vi "PI2_AAN.vi"() -> ()   [LabVIEW 2016]
uses:
  <vilib>/Platform/TimedLoop/XDataNode/nitl_modes.ctl
  <vilib>/Platform/TimedLoop/XDataNode/XDNodeRunTimeDep.lvlib
  <vilib>/Platform/TimedLoop/XDataNode/XDataNode.xnode
  <vilib>/Platform/TimedLoop/XDataNode/timing_clust.ctl
  <vilib>/Platform/TimedLoop/XDataNode/wakeup.ctl
  <vilib>/imath/engines/lvmath2/RunTimeEngine/NodeEndStatement/NIMS_NodeEndStatement_Output.vi
  <vilib>/imath/engines/lvmath2/RunTimeEngine/ErrorHandling/NIMS_Finalize Error.vi
  <vilib>/imath/engines/lvmath2/RunTimeEngine/Managers/WorkSpace/UID Generator.vi
  <vilib>/imath/engines/lvmath2/RunTimeEngine/ArithmeticOperatorToken/NIMS_ArithmeticOperator_times.vi
  <vilib>/imath/engines/lvmath2/RunTimeEngine/BuiltInFunctions/sum/NIMS_sum(GV).vi
  <vilib>/imathl/engines/lvmath/Functions/Error Handling/Create Error.vi
  <vilib>/imath/engines/lvmath2/RunTimeEngine/RangeToken/NIMS_Range.vi
  <vilib>/imath/engines/lvmath2/RunTimeEngine/ArithmeticOperatorToken/NIMS_ArithmeticOperator_plus.vi
  <vilib>/imath/engines/lvmath2/RunTimeEngine/ErrorHandling/NIMS_Create Error From Enums.vi
  <vilib>/imath/engines/lvmath2/RunTimeEngine/BuiltInFunctions/mod/NIMS_mod_no_size_check.vi
  <vilib>/imath/engines/lvmath2/RunTimeEngine/IndexRead/NIMS V(S).vi
  <vilib>/imath/engines/lvmath2/RunTimeEngine/LocalVariableDefStatement/MC_LocalVariableDefStatement_Display.vi
  <vilib>/imath/engines/lvmath2/RunTimeEngine/RunTimeType/NIMS_RunTimeType_From StrictType (excl LVString).vi
  <vilib>/imath/engines/lvmath2/RunTimeEngine/BuiltInFunctions/linramp/NIMS_linramp.vi
  <vilib>/imath/engines/lvmath2/RunTimeEngine/BuiltInFunctions/eye/NIMS_M=eye(I32).vi
  <vilib>/imath/engines/lvmath2/RunTimeEngine/ErrorHandling/NIMS_Error From Error Code.vi
  <vilib>/imath/engines/lvmath2/RunTimeEngine/BuiltInFunctions/zeros/NIMS_V=zeros(I32,I32).vi
  <vilib>/imath/engines/lvmath2/RunTimeEngine/BuiltInFunctions/zeros/NIMS_M=zeros(I32,I32).vi
  <vilib>/imath/engines/lvmath2/RunTimeEngine/IndexReplace/NIMS V(S)=S.vi
  <vilib>/imath/engines/lvmath2/RunTimeEngine/IndexRead/NIMS V(R2).vi
  <vilib>/imath/engines/lvmath2/RunTimeEngine/RangeToken/NIMS_Range_R2 - Float.vi
  <vilib>/imath/engines/lvmath2/RunTimeEngine/IndexRead/NIMS V(V).vi
  <vilib>/imath/engines/lvmath2/RunTimeSupport/NIMS_Error if Not Equal.vi
  <vilib>/imath/engines/lvmath2/RunTimeEngine/ArithmeticOperatorToken/NIMS_ArithmeticOperator_minus.vi
  <vilib>/imath/engines/lvmath2/RunTimeEngine/ArithmeticOperatorToken/NIMS_ArithmeticOperator_power(S).vi
  <vilib>/imath/engines/lvmath2/RunTimeEngine/BuiltInFunctions/abs/NIMS_abs(signed).vi
  <vilib>/imath/engines/lvmath2/RunTimeEngine/CommandStatement/MC_CommandStatement_break.vi
  <vilib>/imath/engines/lvmath2/RunTimeEngine/IndexRead/NIMS M($,S).vi
  <vilib>/imath/engines/lvmath2/RunTimeEngine/IndexReplace/NIMS M($,S)=V.vi
  <vilib>/imath/engines/lvmath2/RunTimeEngine/ArithmeticOperatorToken/NIMS_ArithmeticOperator_multmx(M,CV).vi
  <vilib>/imath/engines/lvmath2/RunTimeEngine/ArithmeticOperatorToken/NIMS_ArithmeticOperator_multmx.vi
  <vilib>/imath/engines/lvmath2/RunTimeEngine/BuiltInFunctions/randnormal/NIMS_randnormal().vi
  <vilib>/imath/engines/lvmath2/RunTimeEngine/BuiltInFunctions/rand/NIMS_rand().vi
  <vilib>/imath/engines/lvmath2/RunTimeEngine/IndexRead/NIMS M($,V).vi
  <vilib>/imath/engines/lvmath2/RunTimeEngine/BuiltInFunctions/sum/NIMS_sum(GM,Sca).vi
  <vilib>/imath/engines/lvmath2/RunTimeEngine/IndexRead/NIMS M(S,S).vi
  <vilib>/imath/engines/lvmath2/RunTimeEngine/IndexReplace/NIMS M($,S)=M.vi
  <vilib>/imath/engines/lvmath2/RunTimeEngine/VariableToken/Support/NIMS_Scalar Boolean Index to I32 Index.vi
  <vilib>/imath/engines/lvmath2/RunTimeEngine/BuiltInFunctions/randnormal/NIMS_randnormal(1,I32).vi
  <vilib>/imath/engines/lvmath2/RunTimeEngine/VariableToken/NIMS_VariableToken_CondDefined.vi
  <vilib>/imath/engines/lvmath2/RunTimeEngine/Managers/SymbolTable/Clear UID.vi
  <vilib>/imath/engines/lvmath2/RunTimeEngine/Managers/SymbolTable/NIMS_WorkSpace.lvlib
  <vilib>/imath/engines/lvmath/Functions/Error Handling/MergeErrorsWrapper.vi
  <vilib>/imath/engines/lvmath2/RunTimeEngine/IndexReplace/NIMS V(V)=S.vi
  <vilib>/imath/engines/lvmath2/RunTimeEngine/IndexReplace/NIMS V(S)=V.vi
  <vilib>/imath/engines/lvmath2/RunTimeEngine/ArithmeticOperatorToken/NIMS_ArithmeticOperator_rightdiv(C,C).vi
  <vilib>/imath/engines/lvmath2/RunTimeEngine/BuiltInFunctions/min/1 input/NIMS_min(CV).vi
  <vilib>/imath/engines/lvmath2/RunTimeEngine/BuiltInFunctions/max/1 input/NIMS_max(CM).vi
  <vilib>/imath/engines/lvmath2/RunTimeEngine/BuiltInFunctions/max/1 input/NIMS_max(CV).vi
  <vilib>/imath/engines/lvmath2/RunTimeEngine/BuiltInFunctions/min/1 input/NIMS_min(CM).vi
  <vilib>/imath/engines/lvmath2/RunTimeEngine/IndexReplace/NIMS M($,S)=S.vi
  <vilib>/imath/engines/lvmath2/RunTimeEngine/IndexReplace/NIMS M(V,S)=V.vi
  <vilib>/imath/engines/lvmath2/RunTimeEngine/IndexReplace/NIMS V(S)=M.vi
  <vilib>/imath/engines/lvmath2/RunTimeEngine/IndexReplace/NIMS M($,V)=M.vi
  <vilib>/imath/engines/lvmath2/RunTimeEngine/ArithmeticOperatorToken/NIMS_ArithmeticOperator_multmx(RV,M).vi
  <vilib>/imath/engines/lvmath2/RunTimeEngine/ArithmeticOperatorToken/NIMS_ArithmeticOperator_rightdivmx.vi
  <vilib>/imath/engines/lvmath2/RunTimeEngine/IndexReplace/NIMS M(S,S)=S.vi
  <vilib>/imath/engines/lvmath2/RunTimeEngine/VariableToken/NIMS_VariableToken_CondDefinedDefinedByReplace.vi
  <vilib>/imath/engines/lvmath2/RunTimeEngine/BuiltInFunctions/inv/NIMS_inv(GM).vi
panel:
  in  "\\lambda_g":dbl
  in  "\\lambda_th":dbl
  in  "\\beta_l":dbl
  in  "\\beta_u":dbl
  in  "\\mu":dbl format="%#_13g"
  in  "?":bool
  in  "M":dbl=4.0 format="%#_13g"
  in  "\\gamma":dbl format="%#_13g"
  out "g":dbl(graph)
  in  "\\sigma":dbl format="%#_13g"
  in  "K":dbl format="%#_13g"
  in  "deadband":dbl format="%#_13g"
  in  "N":dbl format="%#_13g"
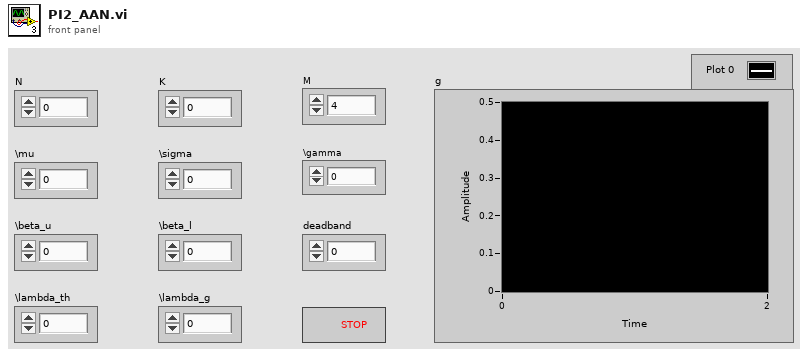
[diagram p1: front panel]
types:
  T1 = typedef "XDNodeRunTimeDep.lvlib/timing_clust.ctl" = cluster{"Expected End [f-1]":u64, "Actual End [f-1]":u64, "Finished Late? [f-1]":bool, "Expected End [i-1]":u64, "Actual End [i-1]":u64, "Finished Late? [i-1]":bool, "Expected Start [i]":u64, "Actual Start [i]":u64, "Expected Start [f]":u64, "Actual Start [f]":u64, "Source Name":string, "Structure Name":string, "Period":i64, "Deadline":i64, "Offset":i64, "Start":i64, "Priority":i32, "Timeout":i32, "Mode":T2, "Wakeup Reason":T3, "Error":errorcluster, "Source Type":string, "Secondary Source Type":string, "Global End Time":u64, "Global Start Time":u64, "Frame Duration":u64, "Iteration Duration":u64, "Assigned CPU":i32, "I/O Scan Engine Mode":u32}
  T2 = typedef "XDNodeRunTimeDep.lvlib/nitl_modes.ctl" = enum32{"No Change", "Process missed periods, maintain original phase", "Discard missed periods, maintain original phase", "Process missed periods, ignore original phase", "Discard missed periods, ignore original phase"}
  T3 = typedef "XDNodeRunTimeDep.lvlib/wakeup.ctl" = enum32{"Normal", "Aborted", "Asynchronous wakeup", "Timing source error", "Timed loop error", "Timeout"}
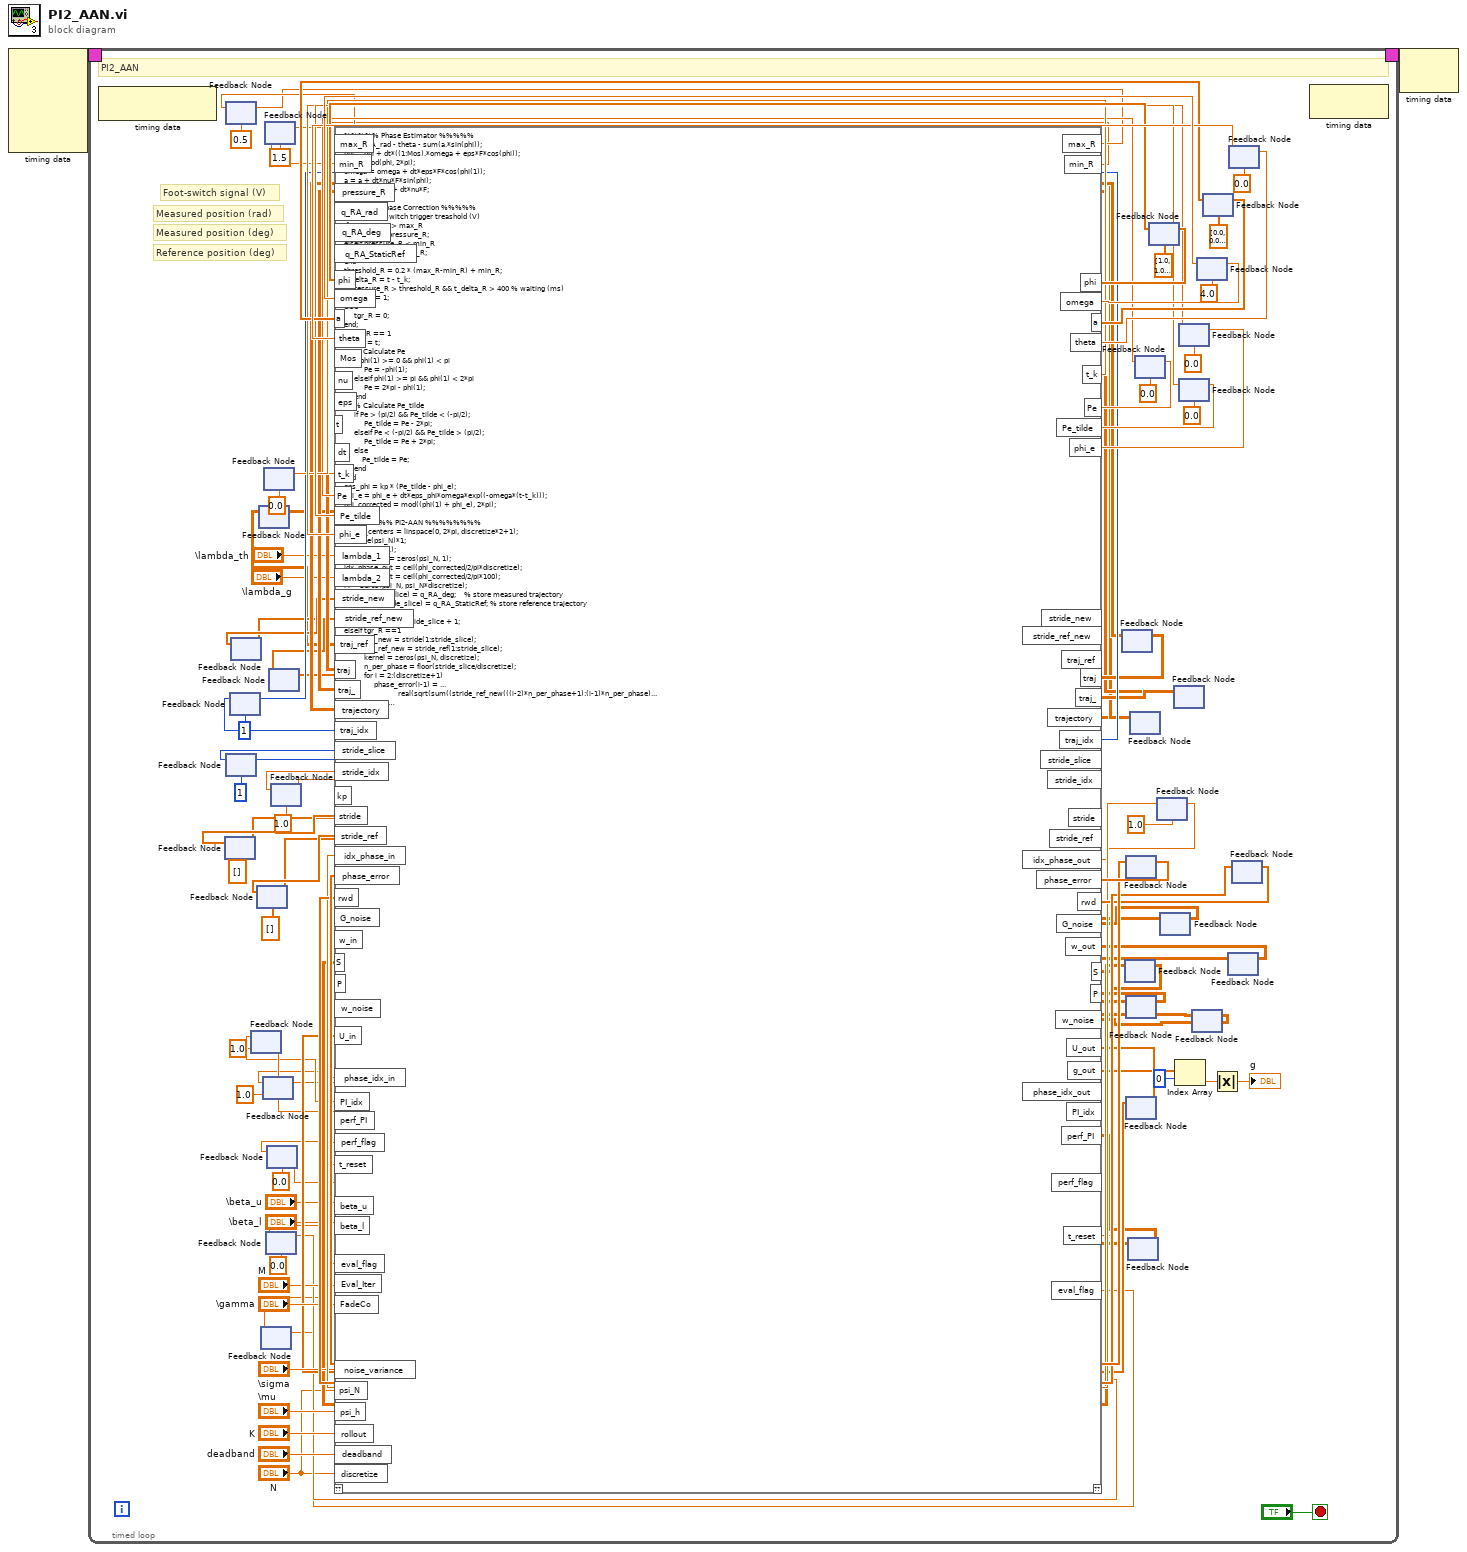
[diagram p0: block diagram]
diagram:
  n1 = node-c288() -> (w2:T1)  [unwired: 5 in]
  n2 = timed-loop {
    timing: w2 -> [_]
    timing-out: [_] -> w1
    stop <- "?" stop-if-true
    # "Reference position (deg)"
    # "Measured position (deg)"
    # "Measured position (rad)"
    # "Foot-switch signal (V)"
    # "PI2_AAN"
    n3 = node-c288() -> ()  [unwired: 1 in, 1 out]
    n4 = feedback #1(dbl[] [] ("stride")) -> (w86:cdb[])
    n5 = feedback #2(0.5 ("max")) -> (w79:dbl)
    n6 = feedback #3(1 ("stride_slice")) -> (w84:i32)
    n7 = feedback #4(1 ("traj_idx")) -> (w71:i32)
    n8 = feedback #5() -> (w24:cdb[])  [unwired: 1 in]
    n9 = feedback #6(1.0 ("PI_idx")) -> (w38:dbl)
    n10 = feedback #7(dbl[] [] ("stride")) -> (w87:cdb[])
    n11 = feedback #8() -> (w17:cdb[][])  [unwired: 1 in]
    n12 = feedback #9() -> (w19:dbl)  [unwired: 1 in]
    n13 = feedback #10(1.0 ("phase_idx_out")) -> (w15:dbl)
    n14 = feedback #11(0.0 ("omega")) -> (w91:dbl)
    n15 = feedback #12(1.5 ("min")) -> (w76:dbl)
    n16 = feedback #13(0.0 ("t_reset")) -> (w30:dbl)
    n17 = feedback #14(0.0 ("perf_flag_ini")) -> (w34:dbl)
    n18 = feedback #15() -> (w23:cdb[])  [unwired: 1 in]
    n19 = feedback #16(1.0 ("stride_idx")) -> (w82:dbl)
    n20 = feedback #17() -> (w69:cdb[][])  [unwired: 1 in]
    n21 = feedback #18() -> (w51:cdb[][])  [unwired: 1 in]
    n22 = feedback #19() -> (w61:cdb[])  [unwired: 1 in]
    n23 = feedback #20() -> (w49:cdb[][])  [unwired: 1 in]
    n24 = feedback #21() -> (w41:cdb[])  [unwired: 1 in]
    n25 = feedback #22() -> (w35:cdb[][])  [unwired: 1 in]
    n26 = feedback #23() -> (w65:cdb[][])  [unwired: 1 in]
    n27 = feedback #24(0.0 ("omega")) -> (w89:dbl)
    n28 = feedback #25(dbl[] [1.0, 1.0, 1.0, 1.0, 1.0, 1.0]) -> (w103:dbl[])
    n29 = feedback #26(1.0 ("idx_phase_out")) -> (w56:dbl)
    n30 = feedback #27() -> (w53:cdb[][])  [unwired: 1 in]
    n31 = feedback #28() -> (w66:cdb[][])  [unwired: 1 in]
    n32 = feedback #29(0.0 ("omega")) -> (w94:dbl)
    n33 = feedback #30(0.0 ("omega")) -> (w97:dbl)
    n34 = feedback #31() -> (w6:cdb[][])  [unwired: 1 in]
    n35 = feedback #32(4.0) -> (w109:dbl)
    n36 = feedback #33(dbl[] [0.0, 0.0, 0.0, 0.0, 0.0, 0.0]) -> (w100:dbl[])
    n37 = feedback #34() -> (w52:cdb[][])  [unwired: 1 in]
    n38 = feedback #35(0.0 ("theta")) -> (w106:dbl)
    n39 = feedback #36() -> (w60:cdb[])  [unwired: 1 in]
    n40 = mathscript code="%%%%% Phase Estimator %%%%%\nF = q_RA_rad - theta - sum(a.*sin(phi));\nphi = phi + dt*((1:Mos).*omega + eps*F*cos(phi));\nphi = mod(phi, 2*pi);\nomega = omega + dt*eps*F*cos(phi(1));\na = a + dt*nu*F*sin(phi);\ntheta = theta + dt*nu*F;\n\n%%%%% Phase Correction %%%%%\n% Find foot-switch trigger treashold (V)\nif pressure_R > max_R\n     max_R = pressure_R;\nelseif pressure_R < min_R\n     min_R = pressure_R;\nend\nthreshold_R = 0.2 * (max_R-min_R) + min_R;\nt_delta_R = t - t_k;\nif pressure_R > threshold_R && t_delta_R > 400 % waiting (ms)\n     tgr_R = 1;\nelse\n     tgr_R = 0;\nend;\nif  tgr_R == 1\n     t_k = t;\n     % Calculate Pe\n     if phi(1) >= 0 && phi(1) < pi\n          Pe = -phi(1);\n     elseif phi(1) >= pi && phi(1) < 2*pi\n          Pe = 2*pi - phi(1);\n     end\n     % Calculate Pe_tilde\n     if Pe > (pi/2) && Pe_tilde < (-pi/2);\n          Pe_tilde = Pe - 2*pi;\n     elseif Pe < (-pi/2) && Pe_tilde > (pi/2);\n          Pe_tilde = Pe + 2*pi;\n     else\n         Pe_tilde = Pe;\n     end    \nend\neps_phi = kp * (Pe_tilde - phi_e);\nphi_e = phi_e + dt*eps_phi*omega*exp((-omega*(t-t_k)));\nphi_corrected = mod((phi(1) + phi_e), 2*pi);\n\n%%%%%%% PI2-AAN %%%%%%%%\nphase_centers = linspace(0, 2*pi, discretize*2+1);\nR = eye(psi_N)*1;\nR_inv = inv(R);\ndelta_w_avg = zeros(psi_N, 1);\nidx_phase_out = ceil(phi_corrected/2/pi*discretize); \nphase_idx_out = ceil(phi_corrected/2/pi*100);\nM = zeros(psi_N, psi_N*discretize);\nstride(stride_slice) = q_RA_deg;    % store measured trajectory \nstride_ref(stride_slice) = q_RA_StaticRef; % store reference trajectory\nif tgr_R ==0\n     stride_slice = stride_slice + 1;\nelseif tgr_R ==1\n     stride_new = stride(1:stride_slice);\n     stride_ref_new = stride_ref(1:stride_slice);\n          kernel = zeros(psi_N, discretize); \n          n_per_phase = floor(stride_slice/discretize);\n          for i = 2:(discretize+1)\n               phase_error(i-1) = ...\n                           real(sqrt(sum((stride_ref_new(((i-2)*n_per_phase+1):(i-1)*n_per_phase)...\n                                                         - stride_new(((i-2)*n_per_phase+1):(i-1)*n_per_phase)).^2)/n_per_phase));\n               % induce deadband\n               phase_error(i-1) = phase_error(i-1)*2;\n               if phase_error(i-1) < deadband\n                    phase_error(i-1) = 0; \n               else\n                    phase_error(i-1) = phase_error(i-1)-deadband;\n               end\n               % compute reward\n               if perf_flag  == 1\n                    lambda_th = lambda_1;\n                    lambda_g = lambda_2;\n               elseif perf_flag == 0;\n                    lambda_th = lambda_2;\n                    lambda_g = lambda_1;\n               end\n               rwd(i-1) = lambda_th*(phase_error(i-1))^2 + lambda_g*(U_in(i-1))^2;\n               for j = 1:psi_N\n                    kernel(j,(i-1)) = exp(-0.5*psi_h*(phase_centers((i-1)*2)-2*pi*(j*2-1)/(psi_N*2))^2);\n               end\n               g_t(:,(i-1)) = kernel(:,(i-1))./sum(kernel(:,(i-1)));\n               M(:,((i-2)*psi_N+1):(i-1)*psi_N) = (R_inv*g_t(:,(i-1))*g_t(:,(i-1))')/(g_t(:,(i-1))'*R_inv*g_t(:,(i-1)));   \n          end\n          perf_sg_stride = real(sqrt(sum((stride_ref_new(floor(stride_slice*0.6):end) - ...\n                                                                       stride_new(floor(stride_slice*0.6):end) ).^2)/(stride_slice*0.4)));\n          % compute roll-out reward S\n          sum_rwd = zeros(discretize,1); wM = zeros(discretize,1);\n          for ii = 1:discretize\n            sum_rwd(ii) = sum(rwd(ii:end));\n            wM(ii) = (w_in + M(:,((ii-1)*psi_N+1):ii*psi_N)*G_noise(:, ((stride_idx-1)*discretize+ii)))'*R*... \n                            (w_in + M(:,((ii-1)*psi_N+1):ii*psi_N)*G_noise(:, ((stride_idx-1)*discretize+ii)));                     \n          end\n          sum_wM = zeros(discretize,1);\n          for jj = 1:discretize\n               sum_wM(jj) = sum(wM(jj+1:end));\n          end\n          S(1:discretize,stride_idx) = sum_rwd + 0.5*sum_wM;\n          % evaluation roll-out flag\n          if eval_flag == 1;\n               perf_PI(:, PI_idx) = perf_sg_stride;\n               PI_idx = PI_idx + 1;\n               if PI_idx > Eval_Iter\n                    PI_idx = 1;\n                    avg_perf_PI = sum(perf_PI)/Eval_Iter;                 \n                    if avg_perf_PI < beta_l\n                         if perf_flag == 0\n                              t_reset = t;\n                         end\n                         perf_flag = 1;\n                    elseif avg_perf_PI >= beta_u\n                         if perf_flag == 1\n                              t_reset = t;\n                         end\n                         perf_flag = 0;\n                    end \n               end\n               stride_idx = 1;\n               eval_flag = 0;  \n          else\n               stride_idx = stride_idx + 1;\n          end\n               if stride_idx > rollout\n                    min_S = min(min(S));\n                    max_S = max(max(S));\n                    stride_idx = 1;\n                    % compute probability P\n                    P_exp = zeros(discretize,rollout);\n                    for i = 1:rollout\n                         P_exp(:,i) = exp(-10*(S(:,i)-min_S)./(max_S-min_S));\n                    end\n                    P_exp_sum = sum(P_exp, 2);\n                    for i = 1:rollout\n                         P(:,i) = P_exp(:,i)./P_exp_sum;\n                    end\n                    % update weights\n                    P_M_e = zeros(psi_N, discretize*rollout);\n                    for j = 1:rollout\n                         for i = 1:discretize\n                              P_M_e(:,((j-1)*discretize+i)) =...\n                              P(i,j)*...\n                              M(:,((i-1)*psi_N+1):i*psi_N)*...\n                              G_noise(:,((j-1)*discretize+i));\n                         end\n                    end\n                    delta_w = zeros(psi_N,discretize); \n                    for i = 1:discretize\n                         tmp = zeros(psi_N,rollout);\n                         for j = 1:rollout\n                              tmp(:,j) = P_M_e(:,((j-1)*discretize+i));\n                         end\n                         delta_w(:,i) = sum(tmp,2);\n                    end\n                    for i = 1:psi_N\n                         delta_w_num = 0; delta_w_den = 0;\n                         for j = 1:discretize\n                              N_kernel = kernel(i,j)*(discretize+1-j);\n                              N_kernel_w = N_kernel*delta_w(i,j);\n                              delta_w_den = delta_w_den + N_kernel;\n                              delta_w_num = delta_w_num + N_kernel_w;\n                         end\n                         delta_w_avg(i) = delta_w_num/delta_w_den;\n                    end \n                    w_out = w_in + delta_w_avg;\n                    eval_flag = 1;\n               end\n          stride_slice = 1;\nend  \n     % add Gaussian noise\n     if (idx_phase_out ~= idx_phase_in) && (eval_flag == 0)\n          fadeout = (FadeCo^(t-t_reset));\n          G_noise(:,((stride_idx-1)*discretize+idx_phase_out)) = sqrt(noise_variance).*randn(psi_N,1)*fadeout;\n     end\n     % generate noisy action\n     if eval_flag == 1\n          w_noise = w_in;\n     else\n          w_noise = w_in + G_noise(:,((stride_idx-1)*discretize+idx_phase_out));\n     end\n     % generate impedance coefficient\n     kernel_output = zeros(psi_N,1);\n     for j = 1:psi_N\n          kernel_output(j) = exp(-0.5*psi_h*(phase_centers(idx_phase_out*2)-2*pi*(j*2-1)/(psi_N*2))^2);\n     end  \n     g_out= sum(kernel_output(:,1).*w_noise)/sum(kernel_output(:,1));\n     U_out(idx_phase_out) = g_out;"("omega"=w109, "theta"=w106, "phi"=w103, "a"=w100, "Pe_tilde"=w97, "phi_e"=w94, "t_k"=w91, "Pe"=w89, "stride_ref"=w87, "stride"=w86, "stride_slice"=w84, "stride_idx"=w82, "max_R"=w79, "min_R"=w76, "traj_idx"=w71, "traj"=w69, "traj_"=w66, "trajectory"=w65, "discretize"="N", "deadband"="deadband", "psi_N"="N", "psi_h"="\\mu", "phase_error"=w61, "rwd"=w60, "rollout"="K", "idx_phase_in"=w56, "noise_variance"="\\sigma", "G_noise"=w53, "w_in"=w52, "S"=w51, "P"=w49, "w_noise"=w6, "U_in"=w41, "FadeCo"="\\gamma", "Eval_Iter"="M", "PI_idx"=w38, "perf_PI"=w35, "perf_flag"=w34, "t_reset"=w30, "stride_new"=w24, "stride_ref_new"=w23, "eval_flag"=w19, "traj_ref"=w17, "phase_idx_in"=w15, "beta_u"="\\beta_u", "beta_l"="\\beta_l", "lambda_1"="\\lambda_th", "lambda_2"="\\lambda_g") -> ("omega"=w110:dbl, "theta"=w107:dbl, "a"=w101:dbl[], "phi"=w104:dbl[], "Pe_tilde"=w98:dbl, "phi_e"=w95:dbl, "t_k"=w92:dbl, "Pe"=w73:dbl, "stride"=w46:cdb[], "stride_ref"=w45:cdb[], "stride_slice"=w85:i32, "stride_idx"=w83:dbl, "max_R"=w78:dbl, "min_R"=w77:dbl, "traj_idx"=w72:i32, "traj"=w68:cdb[][], "traj_"=w67:cdb[][], "trajectory"=w20:cdb[][], "phase_idx_out"=w13:dbl, "phase_error"=w62:cdb[], "rwd"=w59:cdb[], "idx_phase_out"=w25:dbl, "G_noise"=w54:cdb[][], "w_out"=w32:cdb[][], "S"=w50:cdb[][], "P"=w48:cdb[][], "w_noise"=w7:cdb[][], "U_out"=w47:cdb[], "g_out"=w44:cdb[], "PI_idx"=w39:dbl, "perf_PI"=w36:cdb[][], "perf_flag"=w28:dbl, "t_reset"=w31:dbl, "stride_new"=w22:cdb[], "stride_ref_new"=w21:cdb[], "eval_flag"=w16:dbl, "traj_ref"=w18:cdb[][])  [unwired: 11 in, 1 out]
    n41 = feedback-in #1(w46) -> ()
    n42 = feedback-in #2(w78) -> ()
    n43 = feedback-in #3(w85) -> ()
    n44 = feedback-in #4(w72) -> ()
    n45 = feedback-in #5(w22) -> ()
    n46 = feedback-in #6(w39) -> ()
    n47 = feedback-in #7(w45) -> ()
    n48 = feedback-in #8(w18) -> ()
    n49 = feedback-in #9(w16) -> ()
    n50 = feedback-in #10(w13) -> ()
    n51 = feedback-in #11(w92) -> ()
    n52 = feedback-in #12(w77) -> ()
    n53 = feedback-in #13(w31) -> ()
    n54 = feedback-in #14(w28) -> ()
    n55 = feedback-in #15(w21) -> ()
    n56 = feedback-in #16(w83) -> ()
    n57 = feedback-in #17(w68) -> ()
    n58 = feedback-in #18(w50) -> ()
    n59 = feedback-in #19(w62) -> ()
    n60 = feedback-in #20(w48) -> ()
    n61 = feedback-in #21(w47) -> ()
    n62 = feedback-in #22(w36) -> ()
    n63 = feedback-in #23(w20) -> ()
    n64 = feedback-in #24(w73) -> ()
    n65 = feedback-in #25(w104) -> ()
    n66 = feedback-in #26(w25) -> ()
    n67 = feedback-in #27(w54) -> ()
    n68 = feedback-in #28(w67) -> ()
    n69 = Index Array(array=w44, index=0) -> (element=w11:cdb)
    n70 = feedback-in #29(w95) -> ()
    n71 = feedback-in #30(w98) -> ()
    n72 = feedback-in #31(w7) -> ()
    n73 = feedback-in #32(w110) -> ()
    n74 = feedback-in #33(w101) -> ()
    n75 = Absolute Value(x=w11) -> (abs(x)=→"g":dbl)
    n76 = feedback-in #34(w32) -> ()
    n77 = feedback-in #35(w107) -> ()
    n78 = feedback-in #36(w59) -> ()
    n79 = node-c288() -> ()  [unwired: 1 in, 1 out]
  }
  n80 = node-c288(w1) -> ()  [unwired: 1 out]
